vi "Calc_Distance_Angle.vi"(0 "Target Height":dbl=40.5, 1 "Camera Height":dbl=25.0, 2 "X Centroid":dbl, 3 "Y Centroid":dbl, 4 "X Resolution":i32, 5 "Y Resolution":i32, 6 "Half Camera View Angle":dbl=27.0) -> (14 "Shortest Dist To Rect Cent Inches":dbl, 15 "Offset Angle From Perpendicular":dbl)   [LabVIEW 2011]
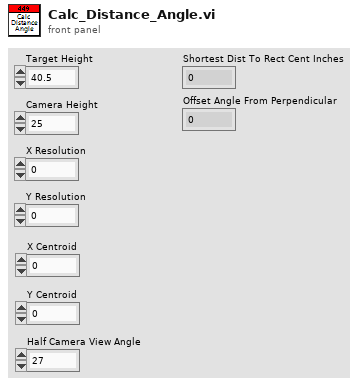
[diagram p1: front panel]
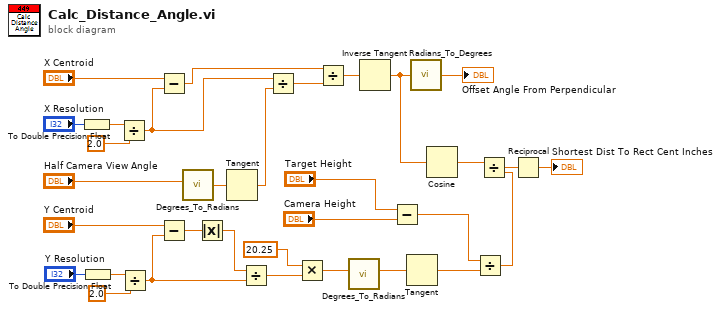
[diagram p0: block diagram]
diagram:
  n1 = To Double Precision Float(number="X Resolution") -> (double precision float=w31:dbl)
  n2 = To Double Precision Float(number="Y Resolution") -> (double precision float=w21:dbl)
  n3 = Divide(x=w31, y=2.0) -> (x/y=w28:dbl)
  n4 = Divide(x=w21, y=2.0) -> (x/y=w19:dbl)
  n5 = Subtract(x="X Centroid", y=w28) -> (x-y=w25:dbl)
  n6 = Subtract(x="Y Centroid", y=w19) -> (x-y=w5:dbl)
  n7 = call "Degrees_To_Radians.vi"("Degrees"="Half Camera View Angle") -> ("Radians"=w29:dbl)  [unwired: 10 in]
  n8 = Absolute Value(x=w5) -> (abs(x)=w4:dbl)
  n9 = Tangent(1:w29) -> (0:w27:dbl)
  n10 = Divide(x=w4, y=w19) -> (x/y=w18:dbl)
  n11 = Divide(x=w28, y=w27) -> (x/y=w26:dbl)
  n12 = Multiply(x=20.25, y=w18) -> (x*y=w2:dbl)
  n13 = Divide(x=w25, y=w26) -> (x/y=w24:dbl)
  n14 = call "Degrees_To_Radians.vi"("Degrees"=w2) -> ("Radians"=w3:dbl)  [unwired: 10 in]
  n15 = Inverse Tangent(1:w24) -> (0:w12:dbl)
  n16 = Subtract(x="Target Height", y="Camera Height") -> (x-y=w14:dbl)
  n17 = Tangent(1:w3) -> (0:w13:dbl)
  n18 = call "Radians_To_Degrees.vi"("Radians"=w12) -> ("Degrees"=→"Offset Angle From Perpendicular":dbl)  [unwired: 10 in]
  n19 = Cosine(x=w12) -> (cos(x)=w11:dbl)
  n20 = Divide(x=w14, y=w13) -> (x/y=w10:dbl)
  n21 = Divide(x=w11, y=w10) -> (x/y=w9:dbl)
  n22 = Reciprocal(x=w9) -> (1/x=→"Shortest Dist To Rect Cent Inches":dbl)
